vi "U8_3_byte_Array_to_voltage_current_Rev03.vi"(0 "Nmbr_of_datapoints":dbl=128.0, 1 "Array In":u8[](array[numeric]), 2 "INPUT1 AC couple":bool, 3 "INPUT2 AC couple":bool, 4 "Div INPUT 2R":dbl, 5 "Div INPUT 1L":dbl, 6 "Shift INPUT 2R":dbl, 7 "Control Character":string, 11 "AC/DC":bool, 12 "Shift INPUT 1L":dbl) -> (8 "INPUT1RMS":dbl, 9 "INPUT2RMS":dbl, 10 "INPUT1 Vave":dbl, 13 "INPUT2 Vave":dbl, 15 "INPUT 1L":dbl[](graph), 16 "INPUT1DC":dbl, 17 "INPUT 2R":dbl[](graph), 19 "INPUT2DC":dbl)   [LabVIEW 2012]
uses:
  <vilib>/measure/madcrms.llb/Basic Averaged DC-RMS for 1 Chan.vi
  <vilib>/Analysis/3filter.llb/Butterworth Filter (DBL).vi
  <vilib>/measure/NI_MAPro.lvlib
  <vilib>/Analysis/NI_AALBase.lvlib
panel:
  out "IPUT2R Line In":dbl[](graph)
  out "INPUT1L Line In":dbl[](graph)
  out "number of samples":dbl
  # "WORK IN PROGRESS"
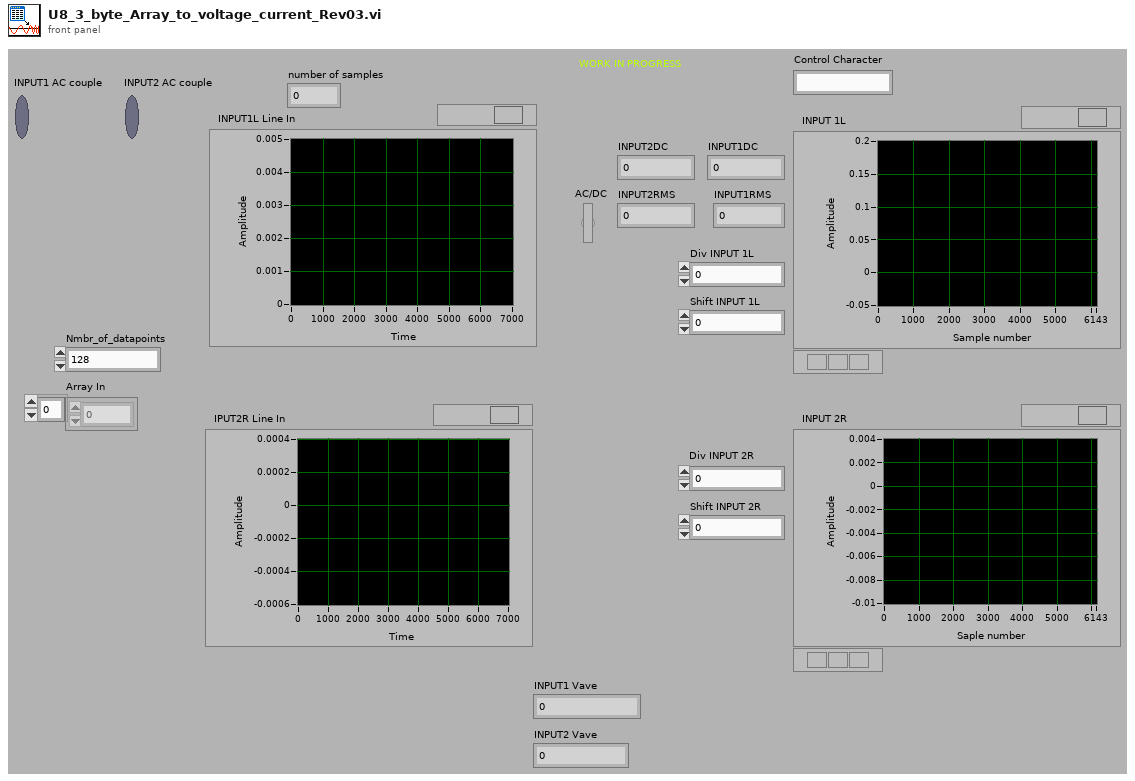
[diagram p1: front panel]
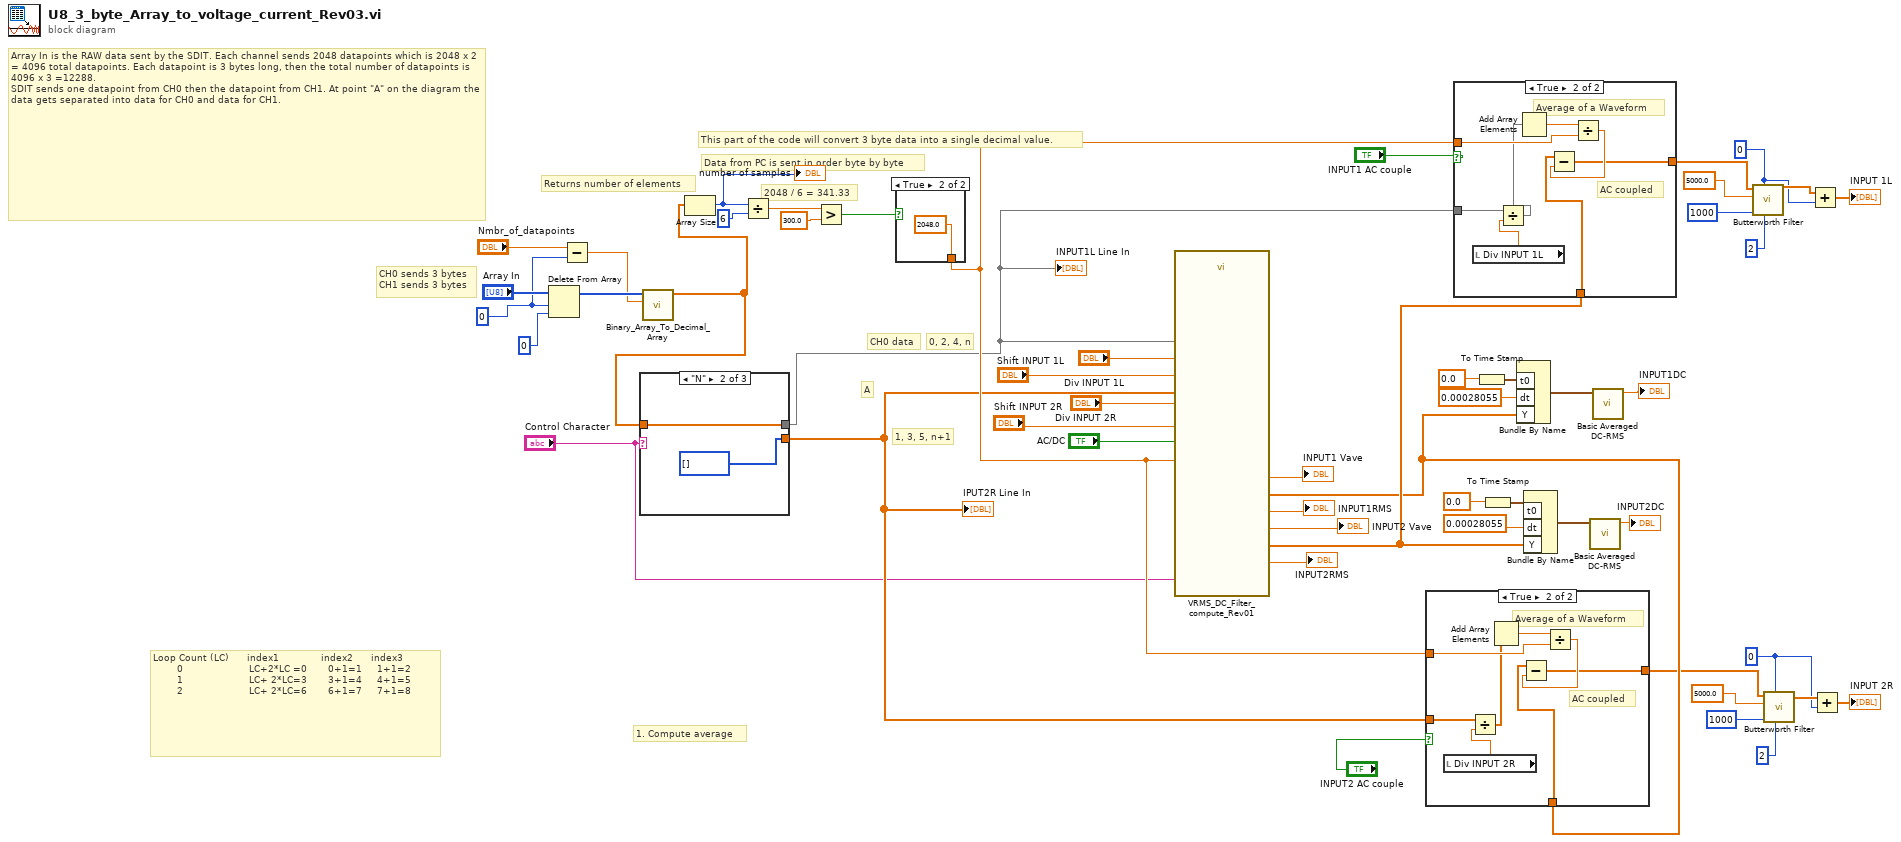
[diagram p0: block diagram]
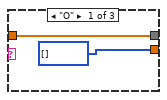
[diagram p2: hidden frame]
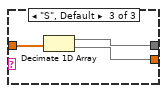
[diagram p3: hidden frame]
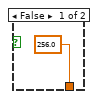
[diagram p6: hidden frame]
diagram:
  w11 = 0
  w12 = 0
  w50 = 0
  # "CH0 data"
  # "A"
  # "Data from PC is sent in order byte by byte"
  # "Array In is the RAW data sent by the SDIT. Each channel sends 2048 datapoints which is 2048 x 2 = 4096 total datapoints. Each datapoint is 3 bytes long, then the total number of datapoints is 4096 x 3 =12288.\nSDIT sends one datapoint from CH0 then the datapoint from CH1. At point \"A\" on the diagram the data gets separated into data for CH0 and data for CH1."
  # "Returns number of elements"
  # "This part of the code will convert 3 byte data into a single decimal value."
  # "2048 / 6 = 341.33"
  # "1. Compute average"
  # "1, 3, 5, n+1"
  # "0, 2, 4, n"
  # "CH0 sends 3 bytes\nCH1 sends 3 bytes"
  # "Loop Count (LC)      index1              index2      index3      \n        0                      LC+2*LC =0       0+1=1     1+1=2\n        1                      LC+ 2*LC=3       3+1=4     4+1=5\n        2                      LC+ 2*LC=6       6+1=7     7+1=8"
  n1 = Delete From Array(array="Array In", length=w50, index=0) -> (array with subset deleted=w6:u8[])  [unwired: 1 out]
  n2 = Subtract(x="Nmbr_of_datapoints", y=w50) -> (x-y=w5:dbl)
  n3 = call "Binary_Array_To_Decimal_Array.vi"("Nmbr_of_datapoints"=w5, "Array In"=w6) -> ("Array Out"=w4:dbl[])  [unwired: 6 in, 3 out]
  n4 = case shown="\"N\"" "Control Character" {
    tunnel: w4 -> [w55 w57 w60]
    tunnel: [w55 w57 w59] -> w3
    tunnel: [i32[] [] i32[] [] w58] -> w2
    frame "O" {
    }
    frame "N" {
    }
    frame "S", Default {
      n5 = Decimate 1D Array(w60) -> (w59:dbl[], w58:dbl[])
    }
  }
  "INPUT1L Line In" <- w3
  "IPUT2R Line In" <- w2
  n6 = Array Size(array=w4) -> (size(s)=w49:i32)
  "number of samples" <- w49
  n7 = Divide(x=w49, y=6) -> (x/y=w48:dbl)
  n8 = Greater?(x=w48, y=300.0) -> (0:w46:bool)
  n9 = case shown="True" w46 {
    tunnel: [256.0 2048.0] -> w21
    frame False {
    }
    frame True {
    }
  }
  n10 = call "VRMS_DC_Filter_compute_Rev01.vi"("INPUT1 Data"=w3, "L Input shift Shift V"="Shift INPUT 1L", "L input multiplier"="Div INPUT 1L", "R Input multiplier"="Div INPUT 2R", "INPUT2 Data"=w2, "Control Character"="Control Character", "DC filter ON/OFF"="AC/DC", "Number Of Samples"=w21, "R Input Shift V"="Shift INPUT 2R") -> ("INPUT1 Vave"=→"INPUT1 Vave":dbl, "INPUT2 Vave"=→"INPUT2 Vave":dbl, "INPUT1RMS"=→"INPUT1RMS":dbl, "INPUT1 Y array"=w18:dbl[], "INPUT2 Y array"=w17:dbl[], "INPUT2RMS"=→"INPUT2RMS":dbl)  [unwired: 1 in]
  n11 = case shown="True" "INPUT2 AC couple" {
    tunnel: w17 -> [w63 w71]
    tunnel: w21 -> [_ w70]
    tunnel: [w63 w67] -> w9
    tunnel: w2 -> [_ w66]
    frame False {
      # "DC coupled"
    }
    frame True {
      # "AC coupled"
      # "Average of a Waveform"
      n12 = local read "Div INPUT 2R"() -> (w65:dbl)
      n13 = Divide(x=w66, y=w65) -> (x/y=w64:dbl[])
      n14 = Add Array Elements(numeric array=w64) -> (sum=w69:dbl)
      n15 = Divide(x=w69, y=w70) -> (x/y=w68:dbl)
      n16 = Subtract(x=w71, y=w68) -> (x-y=w67:dbl[])
    }
  }
  n17 = case shown="True" "INPUT1 AC couple" {
    tunnel: w18 -> [w72 w80]
    tunnel: w21 -> [_ w79]
    tunnel: [w72 w76] -> w10
    tunnel: w3 -> [_ w75]
    frame False {
      # "DC coupled"
    }
    frame True {
      # "AC coupled"
      # "Average of a Waveform"
      n18 = local read "Div INPUT 1L"() -> (w74:dbl)
      n19 = Divide(x=w75, y=w74) -> (x/y=w73:dbl[])
      n20 = Add Array Elements(numeric array=w73) -> (sum=w78:dbl)
      n21 = Divide(x=w78, y=w79) -> (x/y=w77:dbl)
      n22 = Subtract(x=w80, y=w77) -> (x-y=w76:dbl[])
    }
  }
  n23 = To Time Stamp(1:0.0 ("t0")) -> (0:w43:timestamp)
  n24 = To Time Stamp(1:0.0 ("t0")) -> (0:w39:timestamp)
  n25 = Bundle By Name("t0"=w43, "dt"=0.00028055, "Y"=w17) -> (w44:waveform(dbl))  [unwired: 1 in]
  n26 = Bundle By Name("t0"=w39, "dt"=0.00028055, "Y"=w18) -> (w40:waveform(dbl))  [unwired: 1 in]
  n27 = call-poly <vilib>:"Basic Averaged DC-RMS.vi"("signal in"=w40) -> ("DC value"=→"INPUT2DC":dbl)  [unwired: 7 in, 3 out]
  n28 = call-poly <vilib>:"Basic Averaged DC-RMS.vi"("signal in"=w44) -> ("DC value"=→"INPUT1DC":dbl)  [unwired: 7 in, 3 out]
  n29 = call-poly <vilib>:"Butterworth Filter.vi"("order"=2, "filter type"=w12, "low cutoff freq: fl"=1000, "sampling freq: fs"=5000.0, "X"=w10) -> ("Filtered X"=w16:dbl[])  [unwired: 3 in, 1 out]
  n30 = call-poly <vilib>:"Butterworth Filter.vi"("order"=2, "filter type"=w11, "low cutoff freq: fl"=1000, "sampling freq: fs"=5000.0, "X"=w9) -> ("Filtered X"=w14:dbl[])  [unwired: 3 in, 1 out]
  n31 = Add(x=w16, y=w12) -> (x+y=→"INPUT 1L":dbl[])
  n32 = Add(x=w14, y=w11) -> (x+y=→"INPUT 2R":dbl[])
